vi "PCO_SetRecordingState.vi"(8 "error in (no error)":errorcluster {"code" format="%x"}, 10 "wRecState":u16(ring) items=["stop", "run"], 11 "ph":u64) -> (0 "error out":errorcluster {"code" format="%x"}, 2 "ErrorMessage":i32 format="%x", 3 "ph out":u64)   [LabVIEW 2020, in "SDK.lvlib" / "RecordingControl.lvlib"]
doc: "<b>Description:</b>\nThis function sets the Recording State and waits until the state is valid. If the requested state is already set the function will return a warning. If the state cannot be set within one second (+ current frametime for [stop]), the function will return an error.\n\nThe Recording State controls the run state of the camera. If the Recording State is [run], sensor exposure and readout sequences are started depending on current camera settings (trigger mode, acquire mode, external signals…).\nThe Recording State has the highest priority compared to functions like <acq enbl> or exposure trigger.\nWhen the Recording State is set to [stop], sensor exposure and readout sequences are stopped. If the camera is currently in [sensor_readout] state, this readout is finished, before camera run state is changed to [sensor_idle]. If the camera is currently in [sensor_exposing] state, the exposure is cancelled and camera run state is changed immediately to [sensor_idle].\nIn run state [sensor_idle] the camera is running a special idle mode to prevent dark charge accumulation.\n\nIf any camera parameter was changed: before setting the Recording State to [run], the function PCO_ArmCamera must be called. This is to ensure that all settings were correctly and are accepted by the camera.\nIf a successful Recording State [run] command is sent and recording is started, the images from a previous record to the active segment are lost.\n\n<b>Supported camera type:</b>\nAll cameras\n\n<b>Descriptor dependency:</b>\nNone"
uses:
  RecordingControl.lvlib
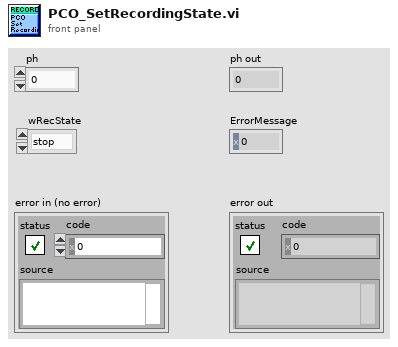
[diagram p1: front panel]
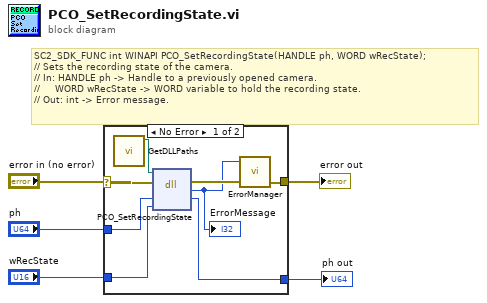
[diagram p0: block diagram]
diagram:
  # "SC2_SDK_FUNC int WINAPI PCO_SetRecordingState(HANDLE ph, WORD wRecState);\n// Sets the recording state of the camera.\n// In: HANDLE ph -> Handle to a previously opened camera.\n//     WORD wRecState -> WORD variable to hold the recording state.\n// Out: int -> Error message."
  n1 = case shown="No Error" "error in (no error)" {
    selector: "error in (no error)" -> [w10 w15]
    tunnel: "ph" -> [w13 w14]
    tunnel: [w12 w14] -> w4
    tunnel: "wRecState" -> [w11 _]
    tunnel: [w8 w15] -> w2
    frame No Error {
      n2 = call "GetDLLPaths.vi"() -> ("SC2_Cam_Path"=w6:path)  [unwired: 9 in, 2 out]
      n3 = dll-call lib="?" fn="PCO_SetRecordingState"(path in=w6, error in=w10, "ph"=w13, "wRecState"=w11) -> (error out=w9:errorcluster, "return type"=w7:i32, "ph"=w12:u64)  [unwired: 2 in, 1 out]
      "ErrorMessage" <- w7
      n4 = call "ErrorManager.vi"("error in (no error)"=w9, "error code"=w7) -> ("error out"=w8:errorcluster)  [unwired: 3 in]
    }
    frame Error {
    }
  }
  "ph out" <- w4
  "error out" <- w2
